vi "Hybrid car new.vi"   [LabVIEW 2016]
uses:
  <vilib>/NXT/Dual Mode Library/Waits/Wait_Num(msec).vi
types:
  T1 = typedef "LVHSConnector.ctl" = refnum<class "BrickReference.lvclass">
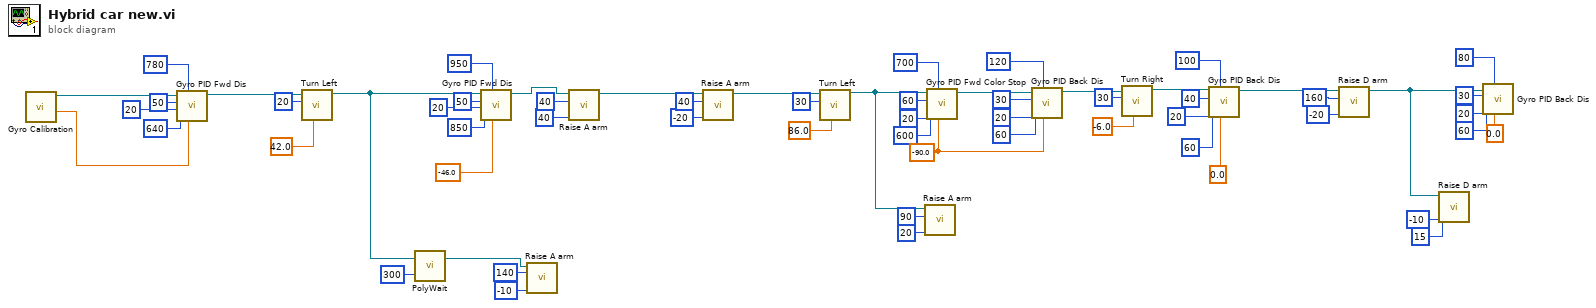
[diagram p0: block diagram]
diagram:
  w21 = sgl -90.0 ("Target angle")
  n1 = call "Gyro Calibration.vi"() -> ("Degrees"=w56:sgl, "NXT/EV3"=w61:T1)  [unwired: 7 in, 1 out]
  n2 = call "Gyro PID Fwd Dis.vi"("Target angle"=w56, "Threshold to stop"=780, "Threshold to slow"=640, "Min. speed"=20, "Max. speed"=50, "EV3 in"=w61) -> ("EV3 out"=w49:T1)  [unwired: 5 in]
  n3 = call "Turn Left.vi"("Turning angle"=sgl 42.0, "Motor B (right)"=i8 20, "EV3 in"=w49) -> ("EV3 out"=w45:T1)  [unwired: 8 in]
  n4 = call-poly <vilib>:"PolyWait.vi"("Time (100 msec)"=u32 300, "NXT/EV3"=w45) -> ("NXT/EV3"=w44:T1)  [unwired: 2 in]
  n5 = call "Gyro PID Fwd Dis.vi"("Target angle"=sgl -46.0, "Threshold to stop"=950, "Threshold to slow"=850, "Min. speed"=20, "Max. speed"=50, "EV3 in"=w45) -> ("EV3 out"=w40:T1)  [unwired: 5 in]
  n6 = call "Raise A arm.vi"("Power"=i8 -10, "Rotation"=140, "EV3 in"=w44) -> ()  [unwired: 8 in, 1 out]
  n7 = call "Raise A arm.vi"("Power"=i8 40, "Rotation"=40, "EV3 in"=w40) -> ("EV3 out"=w39:T1)  [unwired: 8 in]
  n8 = call "Raise A arm.vi"("Power"=i8 -20, "Rotation"=40, "EV3 in"=w39) -> ("EV3 out"=w36:T1)  [unwired: 8 in]
  n9 = call "Turn Left.vi"("Turning angle"=sgl 86.0, "Motor B (right)"=i8 30, "EV3 in"=w36) -> ("EV3 out"=w29:T1)  [unwired: 8 in]
  n10 = call "Raise A arm.vi"("Power"=i8 20, "Rotation"=90, "EV3 in"=w29) -> ()  [unwired: 8 in, 1 out]
  n11 = call "Gyro PID Fwd Color Stop.vi"("Target angle"=w21, "Threshold to Color"=700, "Threshold to slow"=600, "Min. speed"=20, "Max. speed"=60, "EV3 in"=w29) -> ("EV3 out"=w26:T1)  [unwired: 5 in]
  n12 = call "Gyro PID Back Dis.vi"("Target angle"=w21, "Threshold to stop"=120, "Threshold to slow"=60, "Min. speed"=20, "Max. speed"=30, "EV3 in"=w26) -> ("EV3 out"=w20:T1)  [unwired: 5 in]
  n13 = call "Turn Right.vi"("Turning angle"=sgl -6.0, "Motor B (right)"=i8 30, "EV3 in"=w20) -> ("EV3 out"=w17:T1)  [unwired: 8 in]
  n14 = call "Gyro PID Back Dis.vi"("Target angle"=sgl 0.0, "Threshold to stop"=100, "Threshold to slow"=60, "Min. speed"=20, "Max. speed"=40, "EV3 in"=w17) -> ("EV3 out"=w11:T1)  [unwired: 5 in]
  n15 = call "Raise D arm.vi"("Power"=i8 -20, "Rotation"=160, "EV3 in"=w11) -> ("EV3 out"=w3:T1)  [unwired: 8 in]
  n16 = call "Raise D arm.vi"("Power"=i8 -10, "Rotation"=15, "EV3 in"=w3) -> ()  [unwired: 8 in, 1 out]
  n17 = call "Gyro PID Back Dis.vi"("Target angle"=sgl 0.0, "Threshold to stop"=80, "Threshold to slow"=60, "Min. speed"=20, "Max. speed"=30, "EV3 in"=w3) -> ()  [unwired: 5 in, 1 out]
